vi "Options Dialog.vi"(10 "Sequence Context In":refnum<k7>) -> (0 "error out":errorcluster)   [LabVIEW 2020, in "Astemes_CSVReportPlugin.lvlib" / "Options Dialog.lvlib"]
uses:
  Options Dialog.lvlib
  <vilib>/addons/TestStand/_TSUtility.llb/TestStand - Start Modal Dialog (Sequence Context).vi
  <vilib>/addons/TestStand/_TSUtility.llb/TestStand - Get Property Value (String).vi
  <vilib>/addons/TestStand/_TSUtility.llb/TestStand - Set Property Value (String).vi
  <vilib>/addons/TestStand/_TSUtility.llb/TestStand - Set Property Value (Boolean).vi
  <vilib>/addons/TestStand/_TSUtility.llb/TestStand - End Modal Dialog (Sequence Context).vi
panel:
  in  "Cancel":bool
  in  "Commit":bool
  in  "Report Directory":path
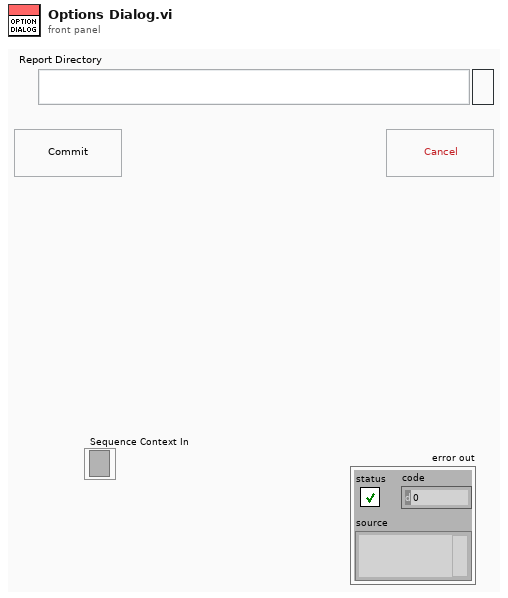
[diagram p1: front panel]
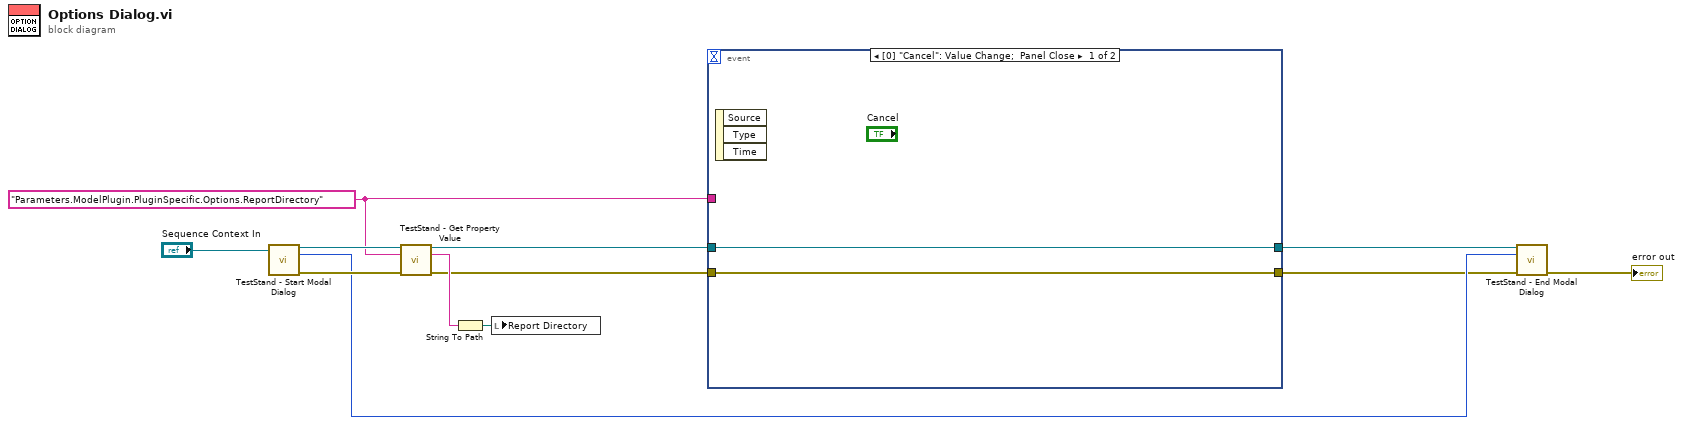
[diagram p0: block diagram]
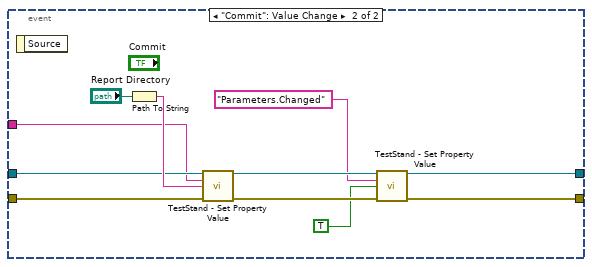
[diagram p2: hidden frame]
diagram:
  w1 = "Parameters.ModelPlugin.PluginSpecific.Options.ReportDirectory" ("Lookup String")
  n1 = call-poly <vilib>:"TestStand - Start Modal Dialog.vi"("Sequence Context In"="Sequence Context In") -> ("Sequence Context Out"=w10:refnum<k7>, "Modal ID"=w6:i32, "error out"=w9:errorcluster)  [unwired: 10 in, 2 out]
  n2 = call-poly <vilib>:"TestStand - Get Property Value.vi"("Sequence Context In"=w10, "Lookup String"=w1, "error in (no error)"=w9) -> ("Sequence Context Out"=w5:refnum<k7>, "Value"=w8:string, "error out"=w4:errorcluster)  [unwired: 10 in]
  n3 = String To Path(string=w8) -> (path=w7:path)
  n4 = local write "Report Directory"(w7) -> ()
  n5 = event shown="[0] \"Cancel\": Value Change;  Panel Close" {
    selector: _ -> [_ _]
    dyn-events: _ -> [_ _]
    timeout: _ -> [_ _]
    tunnel: w5 -> [w13 w23]
    tunnel: w4 -> [w14 w22]
    tunnel: [w14 w18] -> w3
    tunnel: [w13 w19] -> w2
    tunnel: w1 -> [_ w21]
    event "Cancel": Value Change; Panel Close {
      n6 = event-data() -> ()  [unwired: 1 in, 3 out]
    }
    event "Commit": Value Change {
      n7 = event-data() -> ()  [unwired: 1 in, 1 out]
      n8 = Path To String(path="Report Directory") -> (string=w24:string)
      n9 = call-poly <vilib>:"TestStand - Set Property Value.vi"("Sequence Context In"=w23, "Lookup String"=w21, "New Value"=w24, "error in (no error)"=w22) -> ("Sequence Context Out"=w20:refnum<k7>, "error out"=w17:errorcluster)  [unwired: 10 in]
      n10 = call-poly <vilib>:"TestStand - Set Property Value.vi"("Sequence Context In"=w20, "Lookup String"="Parameters.Changed", "New Value"=TRUE, "error in (no error)"=w17) -> ("Sequence Context Out"=w19:refnum<k7>, "error out"=w18:errorcluster)  [unwired: 10 in]
    }
  }
  n11 = call-poly <vilib>:"TestStand - End Modal Dialog.vi"("Sequence Context In"=w2, "Modal ID"=w6, "error in (no error)"=w3) -> ("error out"=→"error out":errorcluster)  [unwired: 12 in]
